vi "LV SciSDK SPECTRUM STOP.vi"(8 "error in (no error)":errorcluster, 9 "Board Handle In":T1, 10 "Spectrum Handle In":T2) -> (0 "error out":errorcluster, 1 "Board Handle Out":T1, 2 "Spectrum Handle Out":T2, 3 "NI Error Code":i32)   [LabVIEW 2021]
uses:
  SciSDK_Labview.lvlib
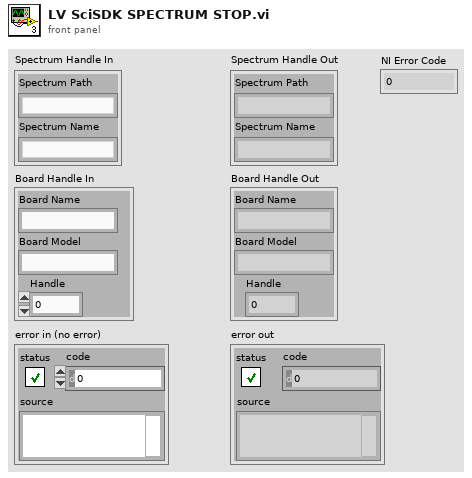
[diagram p1: front panel]
types:
  T1 = cluster{"Board Name":string, "Board Model":string, "Handle":u64}
  T2 = cluster{"Spectrum Path":string, "Spectrum Name":string}
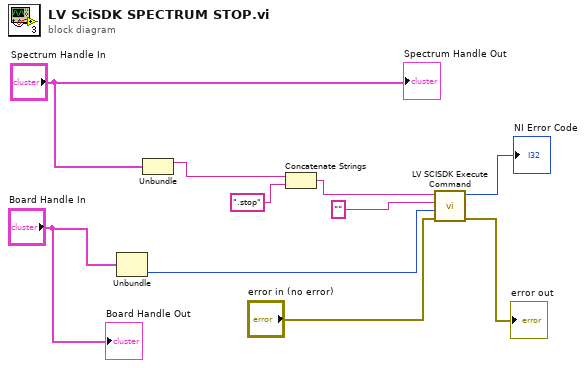
[diagram p0: block diagram]
diagram:
  n1 = Unbundle("Board Handle In") -> ("Handle"=w1:u64)  [unwired: 2 out]
  n2 = Unbundle("Spectrum Handle In") -> ("Spectrum Path"=w3:string)  [unwired: 1 out]
  n3 = Concatenate Strings(w3, ".stop" ("string")) -> (w9:string)
  n4 = call "LV SCISDK Execute Command.vi"("error in (no error)"="error in (no error)", "handle"=w1, "value"="", "Path"=w9) -> ("error out"=→"error out":errorcluster, "function return"=→"NI Error Code":i32)  [unwired: 5 in, 1 out]
  "Spectrum Handle Out" <- "Spectrum Handle In"
  "Board Handle Out" <- "Board Handle In"
